vi "SetValue.vi"(8 "error in":errorcluster, 10 "Value":timestamp, 11 "DateTime in":refnum<class "DateTime.lvclass">) -> (0 "error out":errorcluster, 3 "DateTime out":refnum<class "DateTime.lvclass">)   [LabVIEW 2021, in "ProligentXMLGenerator.lvlib" / "DateTime.lvclass"]
uses:
  DateTime.lvclass
  DateTime.lvclass/DateTime.ctl
  <vilib>/Utility/miscctls.llb/LVDateTimeRec.ctl
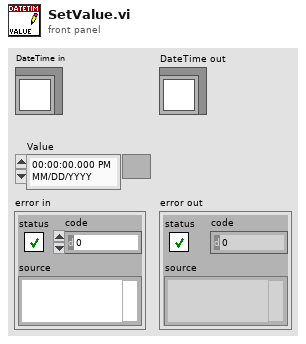
[diagram p1: front panel]
types:
  T1 = typedef "LVDateTimeRec.ctl" = cluster{"fractional second":dbl, "second":i32, "minute":i32, "hour":i32, "day of month":i32, "month":i32, "year":i32, "day of week":i32, "day of year":i32, "DST":i32}
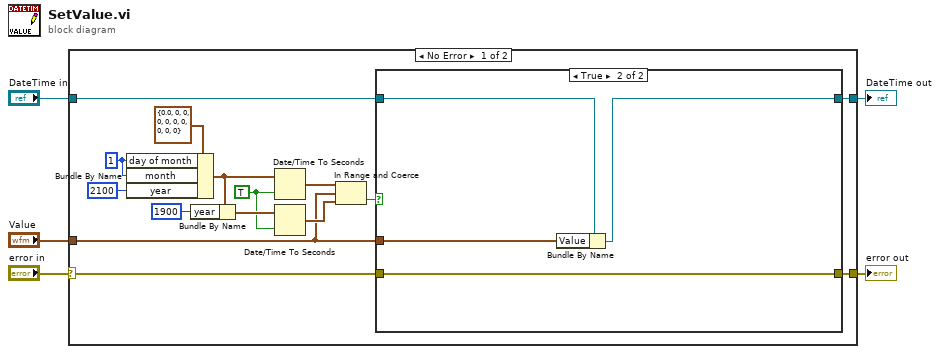
[diagram p0: block diagram]
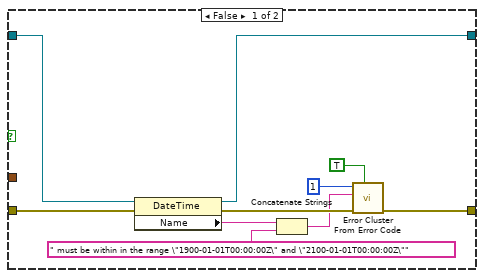
[diagram p2: hidden frame]
diagram:
  n1 = case shown="No Error" "error in" {
    selector: "error in" -> [w6 w35]
    tunnel: [w20 w35] -> w1
    tunnel: [w8 w36] -> w2
    tunnel: "DateTime in" -> [w7 w36]
    tunnel: "Value" -> [w10 _]
    frame No Error {
      w12 = 1 ("day of month")
      w15 = TRUE ("is UTC (F)")
      n2 = Bundle By Name(cluster=T1 {"fractional second"=0.0, "second"=0, "minute"=0, "hour"=0, "day of month"=0, "month"=0, "year"=0, "day of week"=0, "day of year"=0, "DST"=0} ("date time rec"), "day of month"=w12, "month"=w12, "year"=2100) -> (w19:T1)
      n3 = Bundle By Name(cluster=w19, "year"=1900) -> (w18:T1)
      n4 = Date/Time To Seconds(1:w15, 2:w19) -> (0:w17:timestamp)
      n5 = Date/Time To Seconds(1:w15, 2:w18) -> (0:w16:timestamp)
      n6 = In Range and Coerce(upper limit=w17, x=w10, lower limit=w16) -> (In Range?=w9:bool)  [unwired: 1 out]
      n7 = case shown="True" w9 {
        tunnel: w6 -> [w24 w34]
        tunnel: [w29 w34] -> w20
        tunnel: w10 -> [_ w31]
        tunnel: w7 -> [w25 w32]
        tunnel: [w21 w33] -> w8
        frame False {
          n8 = property on="Property Node" class="DateTime"(reference=w25, error in=w24) -> (reference out=w21:refnum<class "DateTime.lvclass">, error out=w23:errorcluster, "Name"=w26:string)
          n9 = Concatenate Strings(w26, " must be within in the range \"1900-01-01T00:00:00Z\" and \"2100-01-01T00:00:00Z\"" ("string")) -> (w22:string)
          n10 = call <vilib>:"Error Cluster From Error Code.vi"("show call chain? (False)"=TRUE, "error in (no error)"=w23, "error message (\"\")"=w22, "error code (0)"=1) -> ("error out"=w29:errorcluster)  [unwired: 5 in]
        }
        frame True {
          n11 = Bundle By Name(cluster=w32, "Value"=w31) -> (w33:refnum<class "DateTime.lvclass">)
        }
      }
    }
    frame Error {
    }
  }
  "error out" <- w1
  "DateTime out" <- w2
